vi "GyroAccel - Standalone Main.vi"() -> ()   [LabVIEW 2021]
uses:
  <vilib>/Platform/TimedLoop/XDataNode/timing_clust.ctl
  <vilib>/Platform/TimedLoop/XDataNode/nitl_modes.ctl
  <vilib>/Platform/TimedLoop/XDataNode/wakeup.ctl
  <vilib>/myRIO/Instrument Drivers/Onboard IO/I2C/typedefs/I2C User Configuration.ctl
  <vilib>/myRIO/Instrument Drivers/Onboard IO/I2C/typedefs/I2C Transfer Rate.ctl
  <vilib>/myRIO/Instrument Drivers/Onboard IO/I2C/typedefs/I2C Reference.ctl
  <vilib>/myRIO/Common/Instrument Driver Framework/Utilities/typedefs/myRIO Generic Hardware Reference.ctl
  <vilib>/myRIO/Common/Instrument Driver Framework/Utilities/typedefs/Hardware Version Enum.ctl
  <vilib>/myRIO/Common/Instrument Driver Framework/Utilities/typedefs/myRIO v1.0 Reference.ctl
  <vilib>/myRIO/Common/Instrument Driver Framework/Utilities/typedefs/Generic FPGA Reference.ctl
  <vilib>/myRIO/Common/Instrument Driver Framework/myRIO v1.0/I2C/typedefs/I2C Channels Enum.ctl
  <vilib>/myRIO/Instrument Drivers/Onboard IO/I2C/typedefs/I2C Configuration.ctl
  <vilib>/userDefined/High Color/nirio_resource_hc.ctl
  <vilib>/myRIO/Common/Instrument Driver Framework/Utilities/vis/Is FPGA Ref Available.vi
  <vilib>/myRIO/Common/Instrument Driver Framework/myRIO v1.0/I2C/vis/myRIO v1.1 Open I2C.vi
  <vilib>/myRIO/Instrument Drivers/Onboard IO/I2C/vis/Configure.vi
  <vilib>/myRIO/Instrument Drivers/Onboard IO/I2C/vis/Write Read.vi
  <vilib>/myRIO/Common/Instrument Driver Framework/Utilities/vis/Validate Channels.vi
  <vilib>/myRIO/Common/Instrument Driver Framework/myRIO v1.0/I2C/vis/myRIO v1.0 Reserve I2C.vi
  <vilib>/myRIO/Common/Instrument Driver Framework/myRIO v1.0/I2C/vis/myRIO v1.0 Build MUX Configuration I2C.vi
  <vilib>/myRIO/Common/Instrument Driver Framework/myRIO v1.0/Resource Manager/vis/myRIO v1.0 Reserve Channel List.vi
  <vilib>/myRIO/Common/Instrument Driver Framework/myRIO v1.0/Resource Manager/vis/myRIO v1.0 Create Configuration List.vi
  <vilib>/myRIO/Common/Instrument Driver Framework/myRIO v1.0/Resource Manager/vis/myRIO v1.0 Reserve Channel.vi
  <vilib>/myRIO/Common/Instrument Driver Framework/myRIO v1.0/Resource Manager/vis/myRIO v1.0 Unreserve Channel.vi
  <vilib>/myRIO/Common/Instrument Driver Framework/myRIO v1.0/Resource Manager/vis/myRIO v1.0 Build Mutex Name.vi
  <vilib>/Utility/VariantDataType/GetNumericInfo.vi
  <vilib>/Utility/error.llb/Error Cluster From Error Code.vi
  <vilib>/myRIO/Common/Instrument Driver Framework/myRIO v1.0/myRIO v1.1 Open.vi
  <vilib>/myRIO/Common/Instrument Driver Framework/Utilities/vis/IO Manager.vi
  <vilib>/myRIO/Common/Instrument Driver Framework/Utilities/vis/Configuration Manager.vi
  <vilib>/myRIO/Common/Instrument Driver Framework/myRIO v1.0/Resource Manager/vis/myRIO v1.0 Configure IO.vi
  <vilib>/myRIO/Common/Instrument Driver Framework/myRIO v1.0/myRIO v1.0 Close.vi
  <vilib>/myRIO/Common/Instrument Driver Framework/myRIO v1.0/I2C/vis/myRIO v1.0 Configure I2C.vi
  <vilib>/myRIO/Common/Instrument Driver Framework/myRIO v1.0/I2C/vis/myRIO v1.0 Write I2C.vi
  <vilib>/myRIO/Common/Instrument Driver Framework/myRIO v1.0/I2C/vis/myRIO v1.0 Read I2C.vi
  <vilib>/platform/TimedLoop/XDataNode/XDataNode.xnode
  <vilib>/myRIO/Express VI/Onboard IO/I2C/I2C Express VI.xnode
  <vilib>/myRIO/Instrument Drivers/Onboard IO/I2C/vis/myRIO I2C Open.xnode
  <vilib>/myRIO/Instrument Drivers/Onboard IO/I2C/I2C.lvlib
  <vilib>/myRIO/Instrument Drivers/Onboard IO/I2C/vis/Write.vi
  <vilib>/Platform/TimedLoop/XDataNode/XDNodeRunTimeDep.lvlib
panel:
  out "Gyro Offset":dbl[](array[numeric])
  in  "initialize":bool
  out "Who Am I":u8[](array[numeric])
  out "Acceleration (g)":T1(graph)
  out "Velocity":T2(graph)
  out "Rotation":T1(graph)
  out "Acceleration (ms^2)":dbl[](array[numeric])
  out "error out":errorcluster
  out "Velocity Cluster Out":cluster{i16, i16, i16}
  out "Rotation Cluster Out":T3
  in  "stop":bool
  in  "error in (no error)":errorcluster
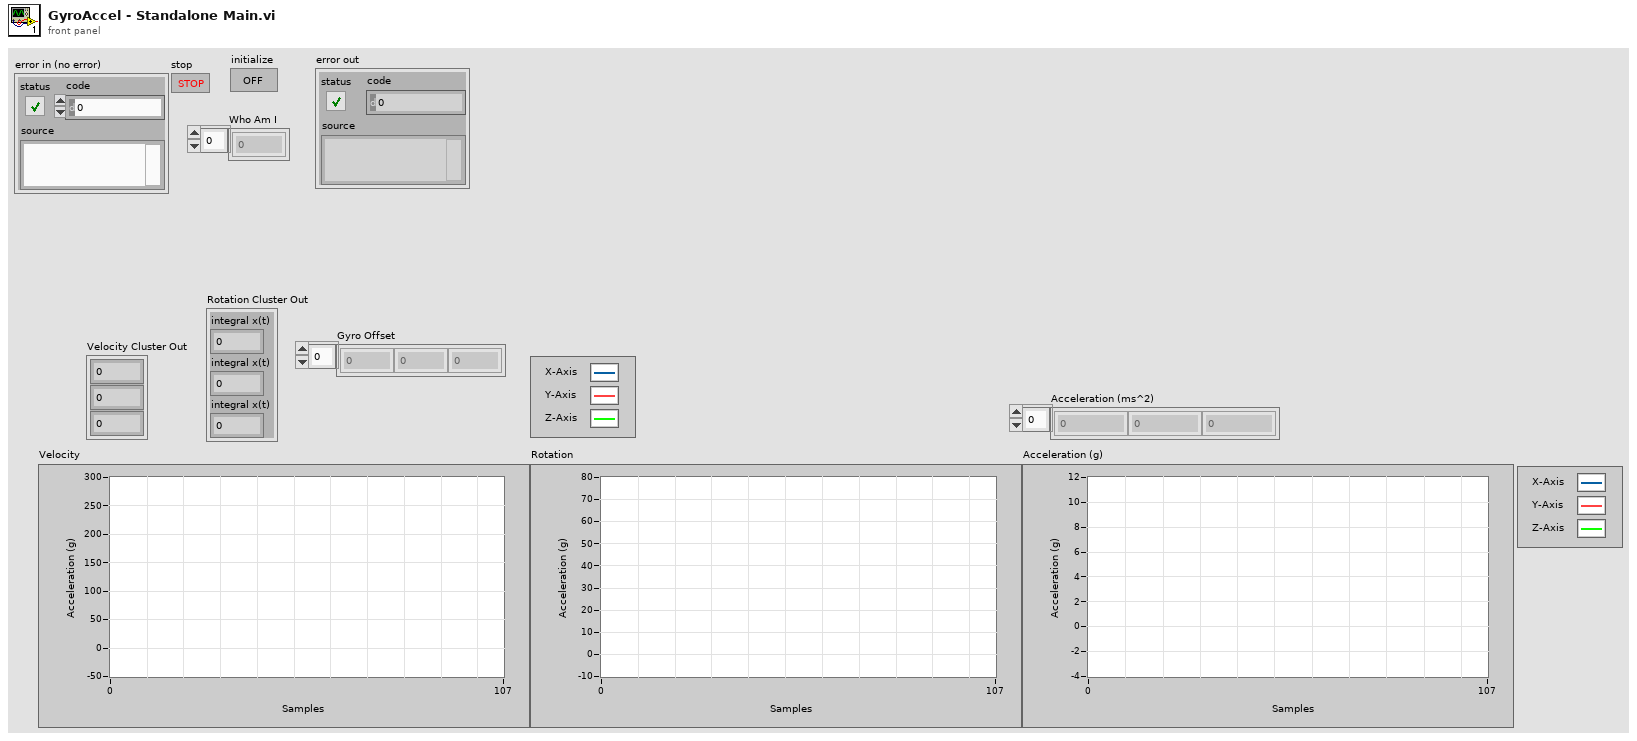
[diagram p1: front panel]
types:
  T1 = cluster{"X-Axis":dbl, "Y-Axis":dbl, "Z-Axis":dbl}
  T2 = cluster{"Velocity":dbl, "Velocity":dbl, "Velocity":dbl}
  T3 = cluster{"integral x(t)":dbl, "integral x(t)":dbl, "integral x(t)":dbl}
  T4 = typedef "I2C.lvlib/I2C Reference.ctl" = cluster{"myRIO Reference":T5, "I2C Channels Enum":T9, "I2C Configuration":T10}
  T5 = typedef "myRIO Generic Hardware Reference.ctl" = cluster{"myRIO Model":T6, "myRIO Hardware Reference":T7}
  T6 = typedef "Hardware Version Enum.ctl" = enum16{"Unknown", "myRIO-1900", "myRIO-1950", "roboRIO", "NI ELVIS RIO CM", "ELVIS III"}
  T7 = typedef "myRIO v1.0 Reference.ctl" = cluster{"Generic FPGA Reference":T8, "Allow multiple opens":bool}
  T8 = typedef "Generic FPGA Reference.ctl" = refnum<k20>
  T9 = typedef "I2C Channels Enum.ctl" = enum16{"Not Connected", "A/I2C", "B/I2C", "I2C/I2C"}
  T10 = typedef "I2C.lvlib/I2C Configuration.ctl" = cluster{"I2C Transfer Rate":T11}
  T11 = typedef "I2C.lvlib/I2C Transfer Rate.ctl" = enum16{"Standard mode (100 kbps)", "Fast mode (400 kbps)"}
  T12 = typedef "I2C.lvlib/I2C User Configuration.ctl" = cluster{"I2C Transfer Rate":T11}
  T13 = typedef "nirio_resource_hc.ctl" = tag
  T14 = typedef "XDNodeRunTimeDep.lvlib/timing_clust.ctl" = cluster{"Expected End [f-1]":u64, "Actual End [f-1]":u64, "Finished Late? [f-1]":bool, "Expected End [i-1]":u64, "Actual End [i-1]":u64, "Finished Late? [i-1]":bool, "Expected Start [i]":u64, "Actual Start [i]":u64, "Expected Start [f]":u64, "Actual Start [f]":u64, "Source Name":string, "Structure Name":string, "Period":i64, "Deadline":i64, "Offset":i64, "Start":i64, "Priority":i32, "Timeout":i32, "Mode":T15, "Wakeup Reason":T16, "Error":errorcluster, "Source Type":string, "Secondary Source Type":string, "Global End Time":u64, "Global Start Time":u64, "Frame Duration":u64, "Iteration Duration":u64, "Assigned CPU":i32, "I/O Scan Engine Mode":u32}
  T15 = typedef "XDNodeRunTimeDep.lvlib/nitl_modes.ctl" = enum32{"No Change", "Process missed periods, maintain original phase", "Discard missed periods, maintain original phase", "Process missed periods, ignore original phase", "Discard missed periods, ignore original phase"}
  T16 = typedef "XDNodeRunTimeDep.lvlib/wakeup.ctl" = enum32{"Normal", "Aborted", "Asynchronous wakeup", "Timing source error", "Timed loop error", "Timeout"}
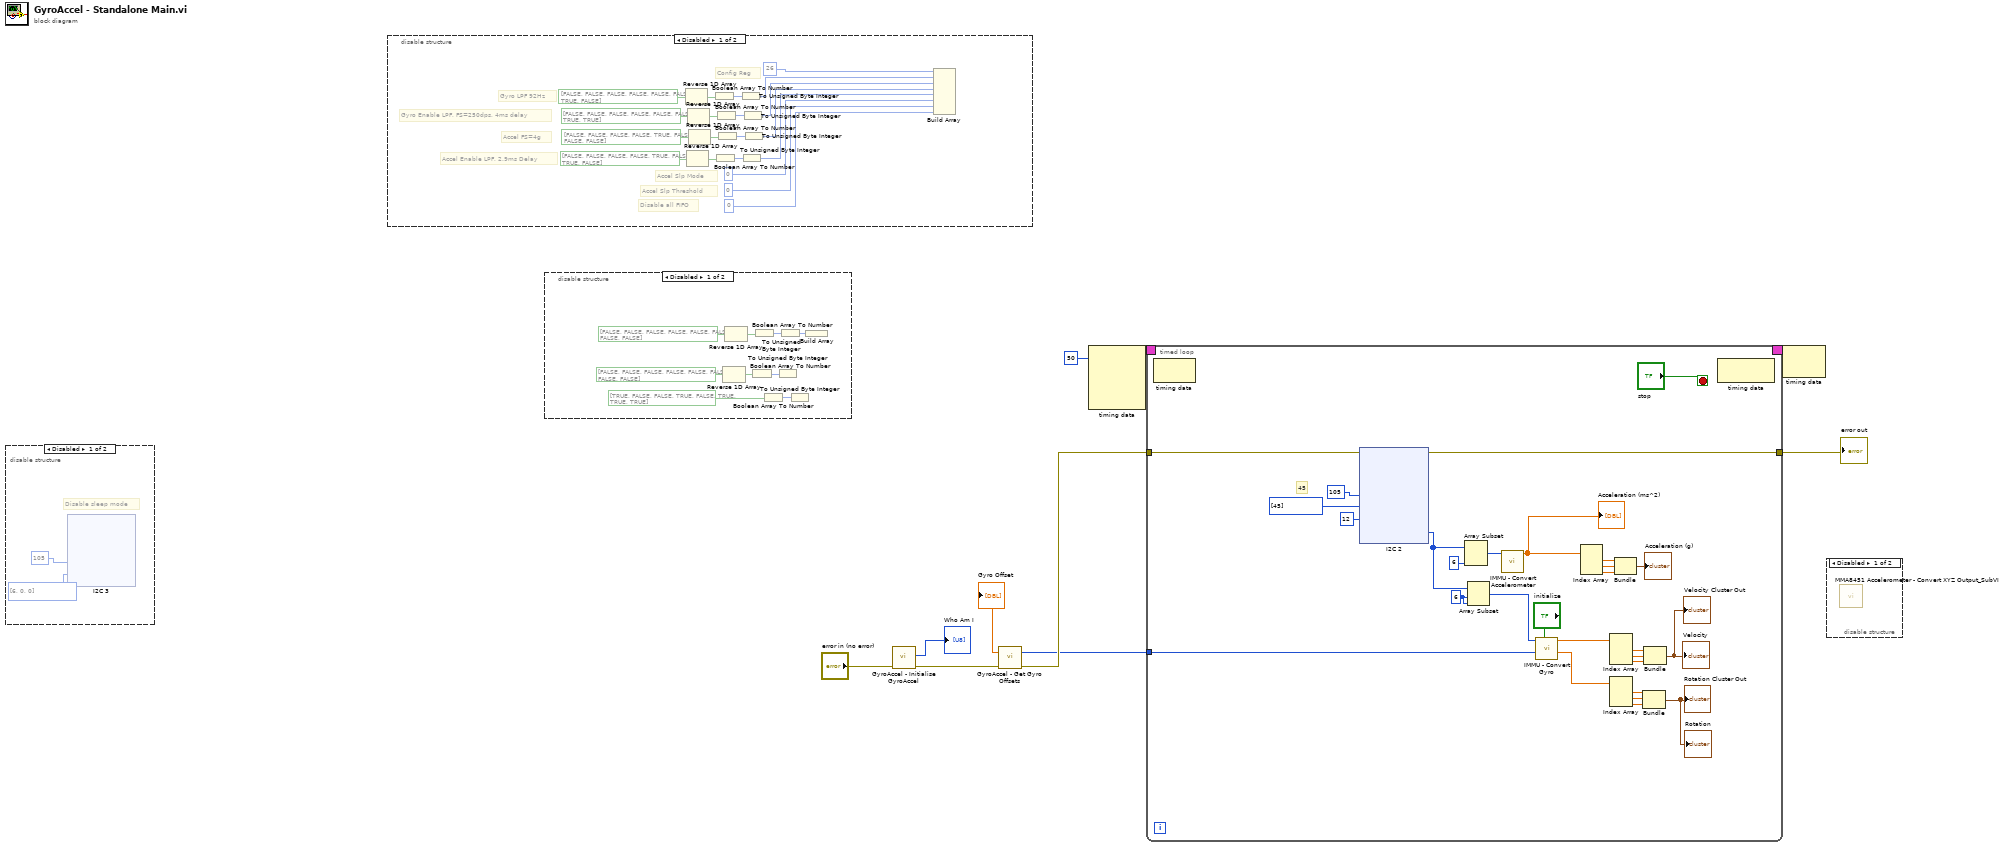
[diagram p0: block diagram]
diagram:
  n1 = disable-structure shown="Disabled" {
    frame Disabled {
      # "Disable sleep mode"
      n2 = xnode "I2C 3"("Slave Address (7-bit)"=u8 105, "Bytes to Write"=u8[] [6, 0, 0]) -> ()  [unwired: 1 in, 1 out]
    }
    frame Enabled {
    }
  }
  n3 = disable-structure shown="Disabled" {
    frame Disabled {
      # "Disable all FIFO"
      # "Accel Slp Threshold"
      # "Accel Slp Mode"
      # "Accel Enable LPF, 2.9ms Delay"
      # "Accel FS=4g"
      # "Gyro LPF 92Hz"
      # "Gyro Enable LPF, FS=250dps, 4ms delay"
      # "Config Reg"
      n4 = Reverse 1D Array(array=bool[] [FALSE, FALSE, FALSE, FALSE, FALSE, FALSE, TRUE, FALSE] ("binary array")) -> (reversed array=w68:bool[])
      n5 = Reverse 1D Array(array=bool[] [FALSE, FALSE, FALSE, FALSE, TRUE, FALSE, TRUE, FALSE] ("binary array")) -> (reversed array=w59:bool[])
      n6 = Reverse 1D Array(array=bool[] [FALSE, FALSE, FALSE, FALSE, FALSE, FALSE, TRUE, TRUE] ("binary array")) -> (reversed array=w65:bool[])
      n7 = Reverse 1D Array(array=bool[] [FALSE, FALSE, FALSE, FALSE, TRUE, FALSE, FALSE, FALSE] ("binary array")) -> (reversed array=w62:bool[])
      n8 = Boolean Array To Number(Boolean array=w68) -> (number=w69:u32)
      n9 = Boolean Array To Number(Boolean array=w59) -> (number=w60:u32)
      n10 = Boolean Array To Number(Boolean array=w65) -> (number=w66:u32)
      n11 = Boolean Array To Number(Boolean array=w62) -> (number=w61:u32)
      n12 = To Unsigned Byte Integer(number=w69) -> (unsigned 8bit integer=w57:u8)
      n13 = To Unsigned Byte Integer(number=w60) -> (unsigned 8bit integer=w54:u8)
      n14 = To Unsigned Byte Integer(number=w66) -> (unsigned 8bit integer=w56:u8)
      n15 = To Unsigned Byte Integer(number=w61) -> (unsigned 8bit integer=w55:u8)
      n16 = Build Array(u8 26 ("Slave Address (7-bit)"), w57, w56, w55, w54, u8 0 ("Slave Address (7-bit)"), u8 0 ("Slave Address (7-bit)"), u8 0 ("Slave Address (7-bit)")) -> ()  [unwired: 1 out]
    }
    frame Enabled {
    }
  }
  n17 = disable-structure shown="Disabled" {
    frame Disabled {
      n18 = Reverse 1D Array(array=bool[] [FALSE, FALSE, FALSE, FALSE, FALSE, FALSE, FALSE, FALSE] ("binary array")) -> (reversed array=w79:bool[])
      n19 = Reverse 1D Array(array=bool[] [FALSE, FALSE, FALSE, FALSE, FALSE, FALSE, FALSE, FALSE] ("binary array")) -> (reversed array=w75:bool[])
      n20 = Boolean Array To Number(Boolean array=w79) -> (number=w78:u32)
      n21 = Boolean Array To Number(Boolean array=w75) -> (number=w76:u32)
      n22 = Boolean Array To Number(Boolean array=bool[] [TRUE, FALSE, FALSE, TRUE, FALSE, TRUE, TRUE, TRUE] ("binary array")) -> (number=w73:u32)
      n23 = To Unsigned Byte Integer(number=w78) -> ()  [unwired: 1 out]
      n24 = To Unsigned Byte Integer(number=w76) -> (unsigned 8bit integer=w71:u8)
      n25 = To Unsigned Byte Integer(number=w73) -> ()  [unwired: 1 out]
      n26 = Build Array(w71) -> ()  [unwired: 1 out]
    }
    frame Enabled {
    }
  }
  n27 = call "GyroAccel - Initialise GyroAccel.vi"("error in (no error)"="error in (no error)") -> ("error out"=w6:errorcluster, "Who Am I"=→"Who Am I":u8[])  [unwired: 8 in, 1 out]
  n28 = call "GyroAccel - Get Gyro Offsets.vi"("error in (no error)"=w6) -> ("error out"=w5:errorcluster, "Output Offset Array"=w2:i16[], "Output Float"=→"Gyro Offset":dbl[])  [unwired: 8 in]
  n29 = node-c288(i64 50 ("Period")) -> (w10:T14)  [unwired: 3 in]
  n30 = timed-loop {
    timing: w10 -> [_]
    timing-out: [_] -> w9
    tunnel: w5 -> [w102]
    tunnel: w2 -> [w97]
    tunnel: [w82] -> w1
    stop <- "stop" stop-if-true
    w84 = 6 ("index")
    # "45"
    n31 = node-c288() -> ()  [unwired: 1 in, 1 out]
    n32 = xnode "I2C 2"("Slave Address (7-bit)"=u8 105, "Bytes to Write"=u8[] [45], "Byte Count"=u32 12, "error in (no error)"=w102) -> ("Bytes Read"=w85:u8[], "error out"=w82:errorcluster)
    n33 = Array Subset(array=w85, length=6) -> (w80:u8[])  [unwired: 1 in]
    n34 = Array Subset(array=w85, index=w84, length=w84) -> (w83:u8[])
    n35 = call "IMMU - Convert Accelerometer.vi"("Input Raw Accel Array (U8)"=w80) -> ("Output Acceleration Array (ms^2)"=w81:dbl[])  [unwired: 10 in]
    "Acceleration (ms^2)" <- w81
    n36 = call "IMMU - Convert Gyro.vi"("initialize"="initialize", "Offset Array In"=w97, "Gyro Data Array In"=w83) -> ("Gyro Rotation Out (degrees)"=w89:dbl[], "Gyro Rotational Velocity Out (deg/s)"=w96:dbl[])  [unwired: 7 in]
    n37 = Index Array(array=w81) -> (element #1=w101:dbl, element #2=w100:dbl, element #3=w99:dbl)  [unwired: 3 in]
    n38 = Index Array(array=w96) -> (element #1=w95:dbl, element #2=w94:dbl, element #3=w93:dbl)  [unwired: 3 in]
    n39 = Index Array(array=w89) -> (element #1=w92:dbl, element #2=w91:dbl, element #3=w90:dbl)  [unwired: 3 in]
    n40 = Bundle(w101, w100, w99) -> (→"Acceleration (g)":cluster{dbl, dbl, dbl})  [unwired: 1 in]
    n41 = Bundle("integral x(t)"=w92, "integral x(t)"=w91, "integral x(t)"=w90) -> (→"Rotation Cluster Out" →"Rotation":T3)  [unwired: 1 in]
    n42 = Bundle(w95, w94, w93) -> (→"Velocity Cluster Out" →"Velocity":cluster{dbl, dbl, dbl})  [unwired: 1 in]
    n43 = node-c288() -> ()  [unwired: 1 in, 1 out]
  }
  "error out" <- w1
  n44 = node-c288(w9) -> ()  [unwired: 1 out]
  n45 = disable-structure shown="Disabled" {
    frame Disabled {
      n46 = call "MMA8451 Accelerometer - Convert XYZ Output_SubVI.vi"() -> ()  [unwired: 11 in, 1 out]
    }
    frame Enabled {
    }
  }
